vi "Configure Sequencer Measurement For Triggering.vi"(8 "error in (no error)":errorcluster, 9 "Measurement For Triggering (\"source\")":string="source", 10 "Instance (1)":i32=1, 11 "VISA resource name":refnum<visa-resource-name>) -> (0 "error out":errorcluster, 3 "VISA resource name out":refnum<visa-resource-name>)   [LabVIEW 2015, in "Rohde&Schwarz CMXP GPRF.lvlib"]
doc: "Selects a measurement for triggering sequencer list incrementations.\n\nAttribute:\nRSCMXPGPRF_ATTR_SEQUENCER_MEASUREMENT_FOR_TRIGGERING\n\nRemote-control command:\nTRIGger:GPRF:GEN<i>:SEQuencer:ISMeas:SOURce"
uses:
  <instrlib>/Rohde&Schwarz CMXP GPRF/Rohde&Schwarz CMXP GPRF.lvlib
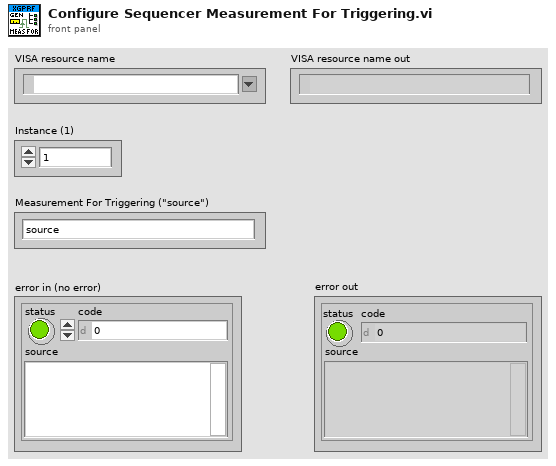
[diagram p1: front panel]
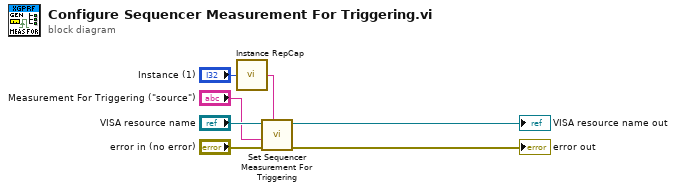
[diagram p0: block diagram]
diagram:
  n1 = call <instrlib>:"Instance RepCap.vi"("instance  in"="Instance (1)") -> ("instance out"=w2:string)
  n2 = call "Set Sequencer Measurement For Triggering"("Repeated Capabilities"=w2, "error in (no error)"="error in (no error)", "Sequencer Measurement For Triggering ()"="Measurement For Triggering (\"source\")", "instrument handle"="VISA resource name") -> ("error out"=→"error out":errorcluster, "instrument handle out"=→"VISA resource name out":refnum<visa-resource-name>)  [unwired: 6 in]
